vi "Perform Action.vi"(8 "error in":errorcluster, 10 "Input":variant, 11 "Virt Instrument Base in":refnum<class "Virt Instr Local.lvclass">) -> (0 "error out":errorcluster, 2 "Output":variant, 3 "Virt Instrument Base out":refnum<class "Virt Instr Local.lvclass">)   [LabVIEW 2023, in "HAL GOOP4.lvlib" / "Virt Instr Local.lvclass"]
uses:
  Virt Instr Local.lvclass
  Virt Instr Local.lvclass/Virt Instr Local.ctl
  Virt Instr Base/Virt Instr Base.lvclass/Virt Instr Base.ctl
  Instrument/Instrument.lvclass
  Virt Instr Base/Virt Instr Base.lvclass
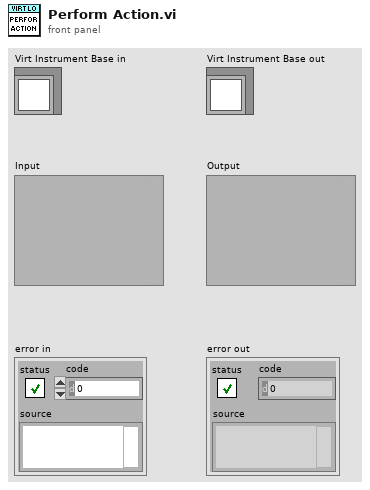
[diagram p1: front panel]
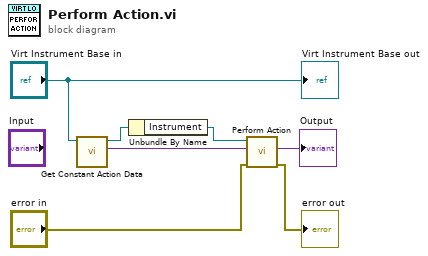
[diagram p0: block diagram]
diagram:
  n1 = call "Get Constant Action Data.vi"("Virt Instr Base in"="Virt Instrument Base in") -> ("Constant Action Data"=w2:variant, "Virt Instr Base out"=w3:refnum<class "Virt Instr Local.lvclass">)  [unwired: 9 in]
  n2 = Unbundle By Name(w3) -> ("Instrument"=w5:refnum<class "Instrument.lvclass">)
  n3 = call "Perform Action.vi"("Error In"="error in", "Input"=w2, "reference in"=w5) -> ("Error Out"=→"error out":errorcluster, "Output"=→"Output":variant)  [unwired: 6 in, 1 out]
  "Virt Instrument Base out" <- "Virt Instrument Base in"
